vi "Get Events.vi"(11 "Series UI Actor in":refnum<class "Series UI Actor.lvclass">) -> (2 "Events":T1, 3 "Series UI Actor out":refnum<class "Series UI Actor.lvclass">)   [LabVIEW 2024, in "Series UI Actor.lvlib" / "Series UI Actor.lvclass"]
uses:
  Series UI Actor.lvclass
  Series UI Actor.lvclass/Series UI Actor.ctl
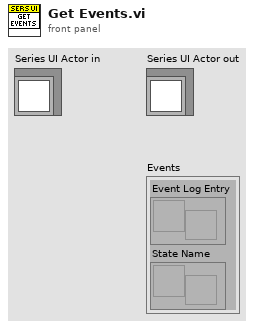
[diagram p1: front panel]
types:
  T1 = cluster{"Event Log Entry":refnum<user-event>, "State Name":refnum<user-event>}
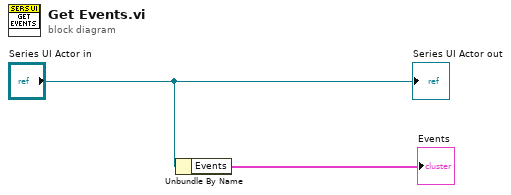
[diagram p0: block diagram]
diagram:
  n1 = Unbundle By Name("Series UI Actor in") -> ("Events"=→"Events":T1)
  "Series UI Actor out" <- "Series UI Actor in"
